vi "TTLsignaldialoge_171213.vi"(0 "Enable":bool=TRUE, 5 "error in (no error)":errorcluster) -> (17 "(in microliter)":dbl format="%#g", 18 "OK":bool, 19 "error out":errorcluster)   [LabVIEW 2016]
doc: "Displays a standard dialog box that prompts users to enter information, such as a user name and password.\n--------------------\n\nThis Express VI is configured as follows:\n\nMessage to Display to the User:How much reward would you like to give?\nThe inputs are: \nNumber: (in microliter)"
panel:
  in  "Tab Control":enum32{"Page 1", "Page 2"}(tab)
  out "String":string="How long is the LED on?"
  in  "OK1":bool
  in  "seconds":dbl caption="(in microliter)" format="%#g"
  in  "Cancel":bool
  in  "OK2":bool
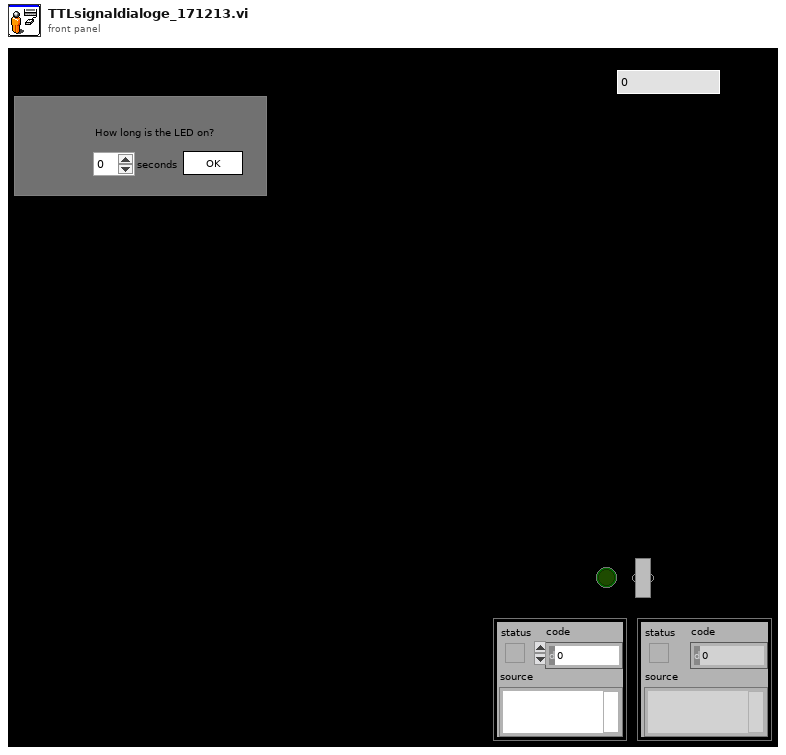
[diagram p1: front panel]
types:
  T1 = cluster{"Input Name":string, "Input Data Type":i32}[]
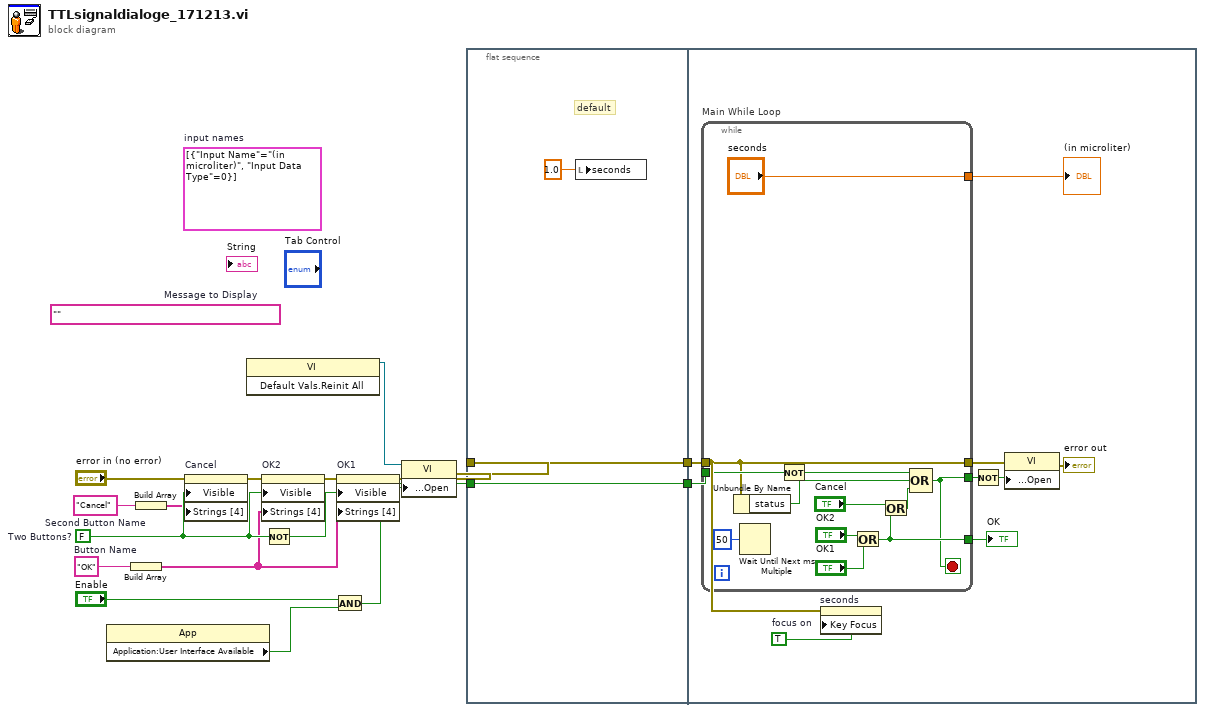
[diagram p0: block diagram]
diagram:
  (unwired) T1 [{"Input Name"="(in microliter)", "Input Data Type"=0}]  # input names
  w12 = "Cancel"  # Second Button Name
  w10 = "OK"  # Button Name
  (unwired) ""  # Message to Display
  w17 = FALSE  # Two Buttons?
  n1 = property class="App"() -> ("Application:User Interface Available"=w4:bool)  [unwired: 2 in, 2 out]
  n2 = Build Array(w10) -> (w11:string[])
  n3 = Build Array(w12) -> (w13:string[])
  n4 = property on="Cancel" class="Bool"(error in="error in (no error)", "Visible"=w17, "Strings [4]"=w13) -> (error out=w15:errorcluster)  [unwired: 1 in, 1 out]
  n5 = invoke class="VI" method="Default Vals.Reinit All"() -> (reference out=w3:refnum<vi>)  [unwired: 3 in, 2 out]
  n6 = property on="OK2" class="Bool"(error in=w15, "Visible"=w17, "Strings [4]"=w11) -> (error out=w14:errorcluster)  [unwired: 1 in, 1 out]
  n7 = Not(x=w17) -> (.not. x?=w16:bool)
  n8 = And(x="Enable", y=w4) -> (x .and. y?=w5:bool)
  n9 = property on="OK1" class="Bool"(error in=w14, "Visible"=w16, "Strings [4]"=w11) -> (error out=w9:errorcluster)  [unwired: 1 in, 1 out]
  n10 = property class="VI"(reference=w3, error in=w9, "Front Panel Window:Open"=w5) -> (error out=w8:errorcluster)  [unwired: 1 out]
  n11 = flat-sequence {
    tunnel: w5 -> [w19]
    tunnel: w8 -> [w20]
    tunnel: [w20] -> w2
    tunnel: [w19] -> w1
    tunnel: w2 -> [w26]
    tunnel: w1 -> [w23]
    frame #0 {
      # "default"
      n12 = local write "seconds"(1.0 ("seconds")) -> ()
    }
    frame #1 {
      w21 = TRUE  # focus on
      n13 = while "Main While Loop" {
        tunnel: [w38] -> w29
        tunnel: w23 -> [w36]
        tunnel: [w34] -> w27
        tunnel: w26 -> [w33]
        tunnel: [w33] -> w25
        tunnel: ["seconds"] -> w22
        stop <- w34 stop-if-true
        n14 = Unbundle By Name(w33) -> ("status"=w31:bool)
        n15 = Wait Until Next ms Multiple(millisecond multiple=u32 50) -> ()  [unwired: 1 out]
        n16 = Not(x=w36) -> (.not. x?=w35:bool)
        n17 = Or(x="OK2", y="OK1") -> (x .or. y?=w38:bool)
        n18 = Or(x="Cancel", y=w38) -> (x .or. y?=w32:bool)
        n19 = Compound Arithmetic op=OR(w35, w31, w32) -> (w34:bool)
      }
      "OK" <- w29
      "(in microliter)" <- w22
      n20 = property on="seconds" class="DigNum (strict)"(error in=w26, "Key Focus"=w21) -> ()  [unwired: 1 in, 2 out]
      n21 = Not(x=w27) -> (.not. x?=w28:bool)
      n22 = property class="VI"(error in=w25, "Front Panel Window:Open"=w28) -> (error out=→"error out":errorcluster)  [unwired: 1 in, 1 out]
    }
  }
